vi "splitInput.vi"(11 "Array in":dbl[](array[numeric])) -> (1 "Amplitude":dbl[](array[numeric]), 2 "Frekvens":dbl[](array[numeric]), 3 "Temperatur":dbl[](array[numeric]), 4 "Perioder":dbl[](array[numeric]))   [LabVIEW 2015]
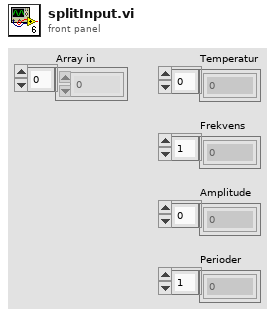
[diagram p1: front panel]
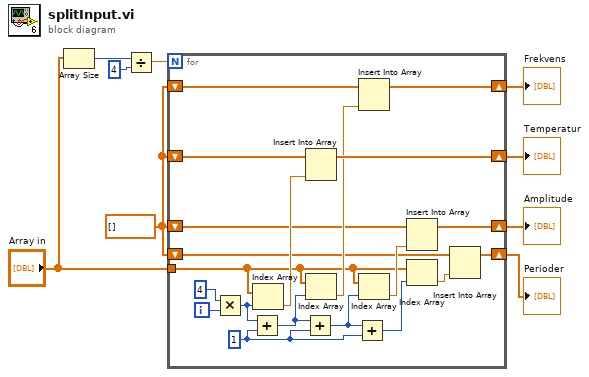
[diagram p0: block diagram]
diagram:
  w7 = dbl[] [] ("Array 2")
  n1 = Array Size(array="Array in") -> (size(s)=w4:i32)
  n2 = Divide(x=w4, y=4) -> (x/y=w5:dbl)
  n3 = for {
    N: w5 -> [_]
    tunnel: "Array in" -> [w16]
    shift-right: [w27] -> w8
    shift-left: w7 -> [w29]
    shift-right: [w25] -> w1
    shift-left: w7 -> [w26]
    shift-right: [w22] -> w2
    shift-left: w7 -> [w23]
    shift-right: [w13] -> w9
    shift-left: w7 -> [w14]
    i -> [w11]
    w18 = 1
    n4 = Multiply(x=4, y=w11) -> (x*y=w10:i32)
    n5 = Add(x=w10, y=w18) -> (x+y=w21:i32)
    n6 = Index Array(array=w16, index=w10) -> (element=w28:dbl)
    n7 = Add(x=w21, y=w18) -> (x+y=w19:i32)
    n8 = Insert Into Array(array=w29, new element=w28) -> (w27:dbl[])  [unwired: 1 in]
    n9 = Index Array(array=w16, index=w21) -> (element=w24:dbl)
    n10 = Add(x=w19, y=w18) -> (x+y=w17:i32)
    n11 = Insert Into Array(array=w26, new element=w24) -> (w25:dbl[])  [unwired: 1 in]
    n12 = Index Array(array=w16, index=w19) -> (element=w20:dbl)
    n13 = Insert Into Array(array=w23, new element=w20) -> (w22:dbl[])  [unwired: 1 in]
    n14 = Index Array(array=w16, index=w17) -> (element=w15:dbl)
    n15 = Insert Into Array(array=w14, new element=w15) -> (w13:dbl[])  [unwired: 1 in]
  }
  "Amplitude" <- w2
  "Perioder" <- w9
  "Temperatur" <- w8
  "Frekvens" <- w1
